vi "SDG60RefClockQ.vi"(2 "error in (no error)":errorcluster, 3 "Ref 10MHz Src (T: Int)":bool=TRUE, 5 "VISA resource name":refnum<visa-resource-name>="USB0::0xF4EC::0x1101::SDG6XEBC5R0119::INSTR") -> (0 "error out":errorcluster, 1 "VISA resource name out":refnum<visa-resource-name>, 4 "String":string="ROSC?")   [LabVIEW 2018]
doc: "Configures the output impedance and source impedance for the channel you specify."
panel:
  # "If no valid external clock present,\noutputs will be switched off"
  # "TODO: output state of\n10 MHz, requires virt keys\nDefault state is off."
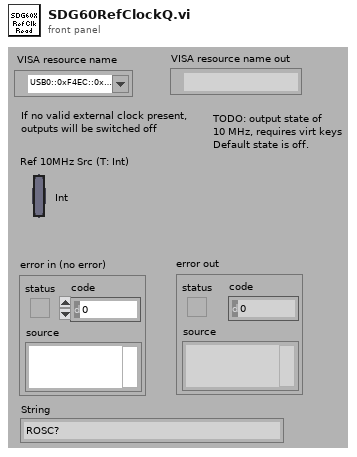
[diagram p1: front panel]
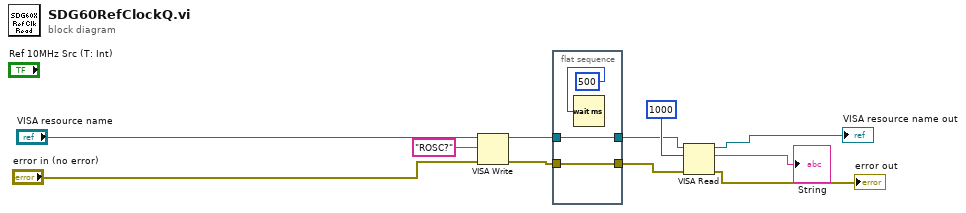
[diagram p0: block diagram]
diagram:
  n1 = VISA Write(VISA resource name="VISA resource name", write buffer="ROSC?", error in (no error)="error in (no error)") -> (VISA resource name out=w5:refnum<visa-resource-name>, error out=w3:errorcluster)  [unwired: 1 out]
  n2 = flat-sequence {
    tunnel: w5 -> [w14]
    tunnel: [w14] -> w4
    tunnel: w3 -> [w13]
    tunnel: [w13] -> w2
    frame #0 {
      n3 = Wait (ms)(milliseconds to wait=500) -> ()  [unwired: 1 out]
    }
  }
  n4 = VISA Read(VISA resource name=w4, byte count=1000, error in (no error)=w2) -> (VISA resource name out=→"VISA resource name out":refnum<visa-resource-name>, read buffer=→"String":string, error out=→"error out":errorcluster)  [unwired: 1 out]
